vi "BRig_dataTrial_DAB_I_flipLR_event.vi"() -> (2 "output_DAB_I_flipLR_event":i32)   [LabVIEW 2014]
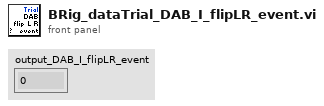
[diagram p1: front panel]
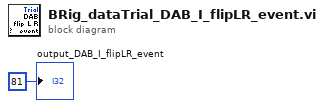
[diagram p0: block diagram]
diagram:
  "output_DAB_I_flipLR_event" <- 81 ("output_iBlock")
